vi "SignalManager.vi"(10 "Signal":T1, 11 "Signal Action":T2) -> (3 "Signal Time":u32)   [LabVIEW 2011]
uses:
  SignalAction.ctl
  Signal.ctl
panel:
  # "Signal Manager stores the time since signal is sent\nI originally implemented it like UNIX signals, where callbacks are registered and sent signals cause callbacks to be called\nI later found that simply receiving a boolean signal output was better, and re-implemented the signal system as it is now"
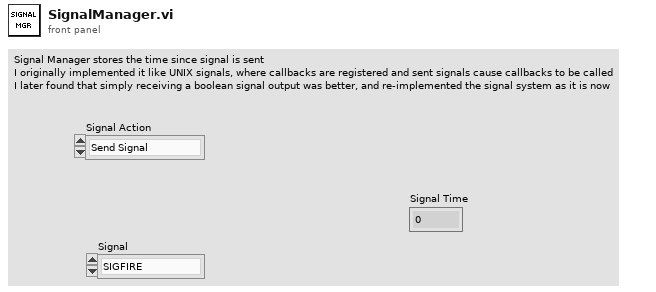
[diagram p1: front panel]
types:
  T1 = typedef "Signal.ctl" = enum16{"SIGFIRE", "SIGSTOPSCRIPT", "SIGSTARTGUN", "SIGSTOPGUN", "SIGDISABLED", "SIGENABLED", "SIGUDPTIMEOUT", "SIGNEWVISION_REMOTE", "SIGNEWVISION_LOCAL", "SIGSHOTFIRED", "SIGDOTRACK", "SIGDONTTRACK"}
  T2 = typedef "SignalAction.ctl" = enum16{"Send Signal", "Get Signal Trap"}
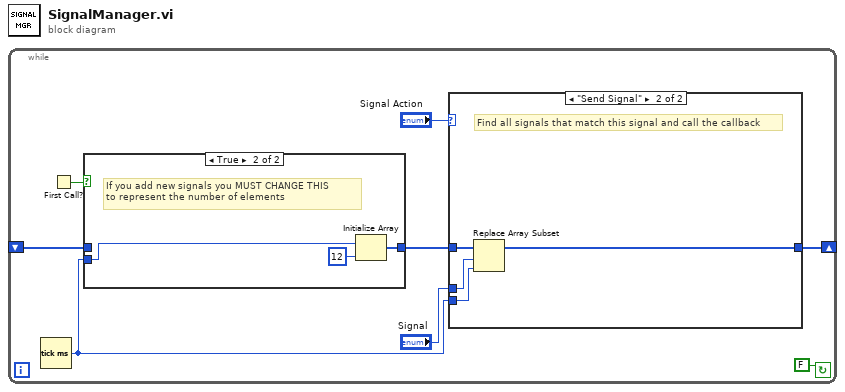
[diagram p0: block diagram]
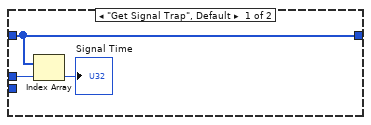
[diagram p3: hidden frame]
diagram:
  n1 = while {
    shift-right: [w5] -> _
    shift-left: _ -> [w2]
    stop <- FALSE continue-if-true
    n2 = Tick Count (ms)() -> (millisecond timer value=w1:u32)
    n3 = First Call?() -> (First Call?: T/F=w4:bool)
    n4 = case shown="True" w4 {
      tunnel: [w9 w11] -> w3
      tunnel: w2 -> [w9 _]
      tunnel: w1 -> [_ w12]
      frame False {
      }
      frame True {
        # "If you add new signals you MUST CHANGE THIS\nto represent the number of elements"
        n5 = Initialize Array(w12, 12 ("dimension size")) -> (w11:u32[])
      }
    }
    n6 = case shown="\"Send Signal\"" "Signal Action" {
      tunnel: "Signal" -> [w15 w17]
      tunnel: w3 -> [w14 w19]
      tunnel: [w14 w18] -> w5
      tunnel: w1 -> [_ w16]
      frame "Get Signal Trap", Default {
        n7 = Index Array(array=w14, index=w15) -> (element=→"Signal Time":u32)
      }
      frame "Send Signal" {
        # "Find all signals that match this signal and call the callback"
        n8 = Replace Array Subset(array=w19, new element=w16, index=w17) -> (w18:u32[])
      }
    }
  }
